vi "2DGraphSetupArrDev.vi"(8 "error in (no error)":errorcluster caption="entrée d'erreur (pas d'erreur)", 11 "Interface en entrée":refnum<class "Interface.lvclass"> caption="DNL_LabVIEW Object in") -> (0 "error out":errorcluster caption="sortie d'erreur", 3 "Interface en sortie":refnum<class "Interface.lvclass"> caption="DNL_LabVIEW Object out")   [LabVIEW 2019, in "Interface.lvclass"]
uses:
  Interface.lvclass
  Experiment Class/Experiment.lvclass
  <userlib>/GenProg/ArrayTo1DString.vi
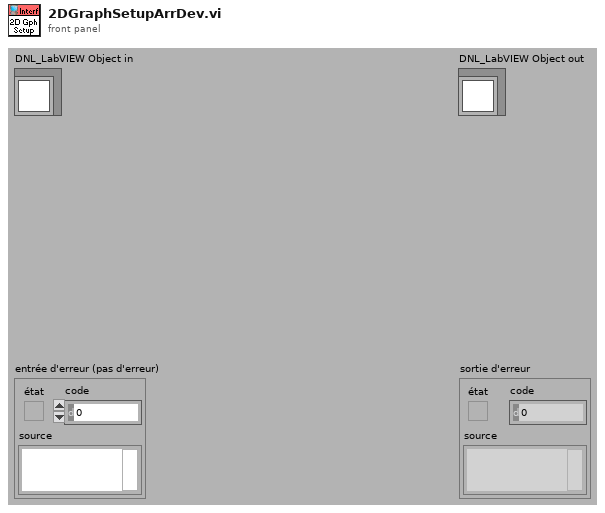
[diagram p1: front panel]
types:
  T1 = typedef "2DGraphSetup.ctl" = cluster{"ZDataIndex":i32, "XParIndex":i32, "YParIndex":i32, "FillLineFirst":bool, "2DGraphIndex":i32, "XParQ Ref":refnum<queue>, "YParQ Ref":refnum<queue>, "DataQRefs":refnum<queue>[], "CurveName":string, "XparInstrInd":i32, "YparInstrInd":i32, "Active":bool}
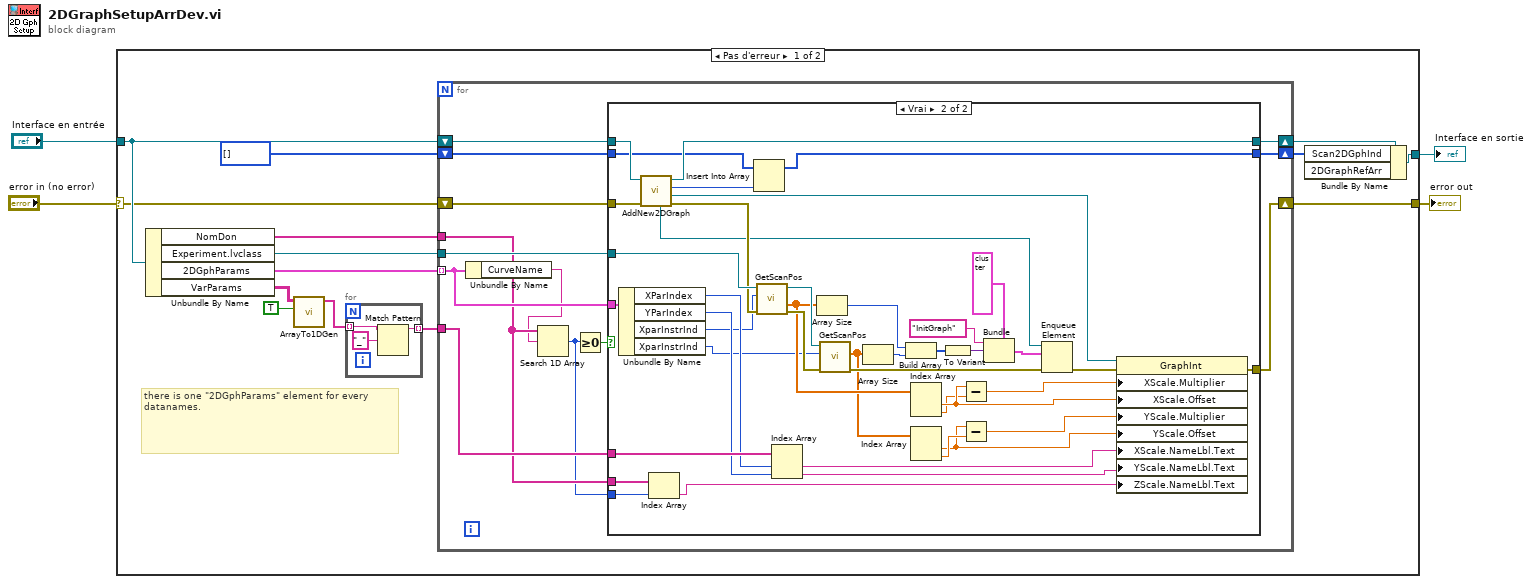
[diagram p0: block diagram]
diagram:
  n1 = case shown="Pas d'erreur" "error in (no error)" {
    selector: "error in (no error)" -> [w12 w80]
    tunnel: [w10 w80] -> w3
    tunnel: [w15 w79] -> w1
    tunnel: "Interface en entrée" -> [w18 w79]
    frame No Error {
      # "there is one \"2DGphParams\" element for every datanames."
      n2 = Unbundle By Name(w18) -> ("NomDon"=w6:string[], "Experiment.lvclass"=w17:refnum<class "Experiment.lvclass">, "2DGphParams"=w11:T1[], "VarParams"=w9:string[][])
      n3 = call-poly <userlib>:"ArrayTo1DGen.vi"("DelArrEnd"=TRUE, "tableau"=w9) -> ("Array Out"=w5:string[])  [unwired: 7 in, 2 out]
      n4 = for {
        tunnel: w5 -> [w21] mode=indexing
        tunnel: [w20] -> w7 mode=indexing
        n5 = Match Pattern(string=w21, regular expression="_" ("expression régulière")) -> (before substring=w20:string)  [unwired: 1 in, 3 out]
      }
      n6 = for {
        tunnel: w11 -> [w34] mode=indexing
        shift-right: [w32] -> w16
        shift-left: w18 -> [w33]
        tunnel: w17 -> [w31]
        shift-right: [w30] -> w14
        shift-left: i32[] [] -> [w29]
        shift-right: [w28] -> w10
        shift-left: w12 -> [w27]
        tunnel: w7 -> [w26]
        tunnel: w6 -> [w25]
        n7 = Unbundle By Name(w34) -> ("CurveName"=w24:string)
        n8 = Search 1D Array(1D array=w25, element=w24) -> (index of element=w23:i32)  [unwired: 1 in]
        n9 = Greater Or Equal To 0?(x=w23) -> (x >= 0?=w22:bool)
        n10 = case shown="Vrai" w22 {
          tunnel: w34 -> [_ w76]
          tunnel: w33 -> [w37 w78]
          tunnel: [w37 w77] -> w32
          tunnel: w31 -> [_ w72]
          tunnel: [w36 w75] -> w30
          tunnel: w29 -> [w36 w73]
          tunnel: [w35 w53] -> w28
          tunnel: w27 -> [w35 w52]
          tunnel: w26 -> [_ w47]
          tunnel: w25 -> [_ w41]
          tunnel: w23 -> [_ w42]
          frame False {
          }
          frame True {
            n11 = Unbundle By Name(w76) -> ("XParIndex"=w45:i32, "YParIndex"=w44:i32, "XparInstrInd"=w39:i32, "XparInstrInd"=w38:i32)
            n12 = call "AddNew2DGraph.vi"("error in (no error)"=w52, "Interface en entrée"=w78) -> ("error out"=w51:errorcluster, "Graph"=w71:refnum<vi>, "NewGraphInd"=w74:i32, "Interface en sortie"=w77:refnum<class "Interface.lvclass">, "2DGraphQRef"=w49:refnum<queue>)  [unwired: 5 in]
            n13 = Index Array(array=w41, index=w42) -> (element=w40:string)
            n14 = Insert Into Array(array=w73, new element=w74) -> (w75:i32[])  [unwired: 1 in]
            n15 = call "GetScanPos.vi"("error in (no error)"=w51, "ParIndex"=w39, "Experiment en entrée"=w72) -> ("error out"=w67:errorcluster, "ScanTable"=w59:dbl[], "Experiment en sortie"=w68:refnum<class "Experiment.lvclass">)  [unwired: 6 in]
            n16 = Index Array(array=w47, index #1=w45, index #2=w44) -> (element #1=w46:string, element #2=w43:string)
            n17 = Array Size(array=w59) -> (size(s)=w70:i32)
            n18 = call "GetScanPos.vi"("error in (no error)"=w67, "ParIndex"=w38, "Experiment en entrée"=w68) -> ("error out"=w65:errorcluster, "ScanTable"=w55:dbl[])  [unwired: 6 in, 1 out]
            n19 = Array Size(array=w55) -> (size(s)=w69:i32)
            n20 = Build Array(w70, w69) -> (w62:i32[])
            n21 = Index Array(array=w59) -> (element #1=w58:dbl, element #2=w57:dbl)  [unwired: 2 in]
            n22 = Index Array(array=w55) -> (element #1=w48:dbl, element #2=w50:dbl)  [unwired: 2 in]
            n23 = To Variant(anything=w62) -> (Variant=w61:variant)
            n24 = Subtract(x=w58, y=w57) -> (x-y=w56:dbl)
            n25 = Subtract(x=w48, y=w50) -> (x-y=w54:dbl)
            n26 = Bundle(cluster=cluster{"Message":string, "Data":variant, i32} {"Message"="", "Data"=variant, 0} ("élément"), "Message"="InitGraph", "Data"=w61) -> (w64:cluster{"Message":string, "Data":variant, i32})  [unwired: 1 in]
            n27 = Enqueue Element(queue=w49, element=w64, error in (no error)=w65) -> (error out=w60:errorcluster)  [unwired: 1 in, 2 out]
            n28 = property class="GraphInt"(reference=w71, error in=w60, "XScale.Multiplier"=w56, "XScale.Offset"=w58, "YScale.Multiplier"=w54, "YScale.Offset"=w48, "XScale.NameLbl.Text"=w46, "YScale.NameLbl.Text"=w43, "ZScale.NameLbl.Text"=w40) -> (error out=w53:errorcluster)  [unwired: 1 out]
          }
        }
      }
      n29 = Bundle By Name(cluster=w16, "Scan2DGphInd"=w14) -> (w15:refnum<class "Interface.lvclass">)  [unwired: 1 in]
    }
    frame Error {
    }
  }
  "error out" <- w3
  "Interface en sortie" <- w1
